vi "test.2dArrays.vi"(8 "error in":errorcluster, 10 "Data":variant, 11 "Command":string) -> (0 "error out":errorcluster, 3 "Return Data":variant)   [LabVIEW 2014]
uses:
  Private/Class/meth.Constructor.vi
  Private/Class/meth.Destructor.vi
  GLue.lvlib
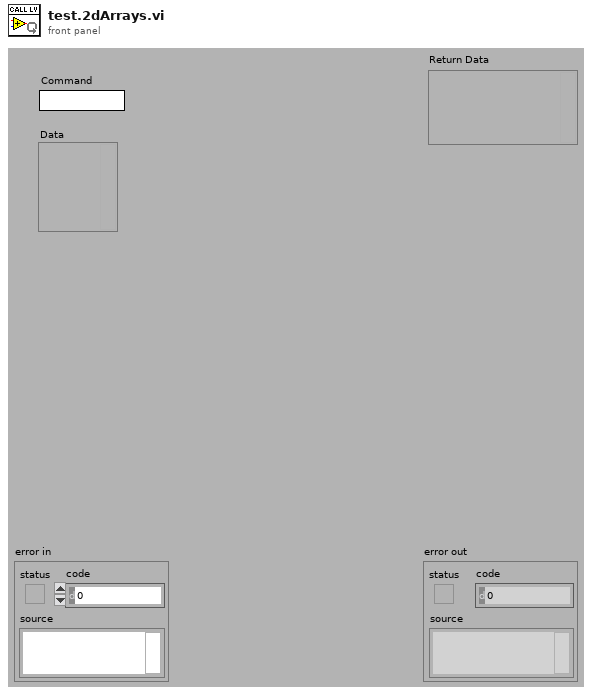
[diagram p1: front panel]
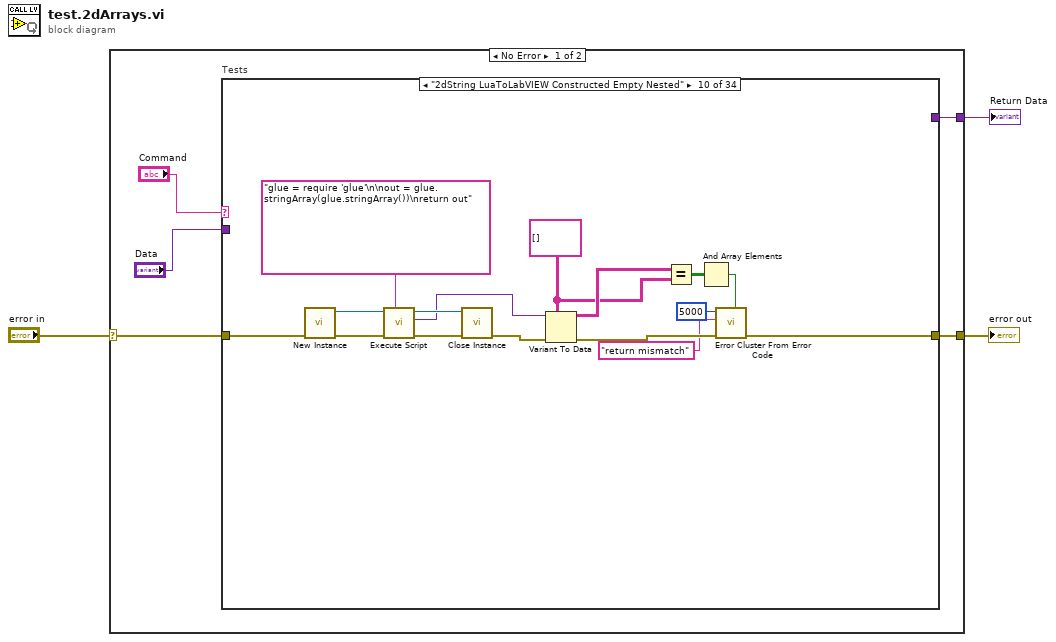
[diagram p0: block diagram]
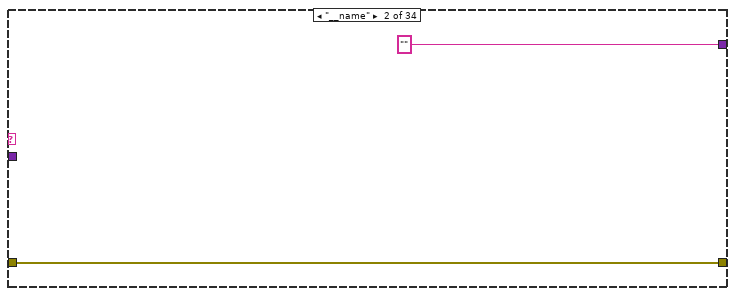
[diagram p3: hidden frame]
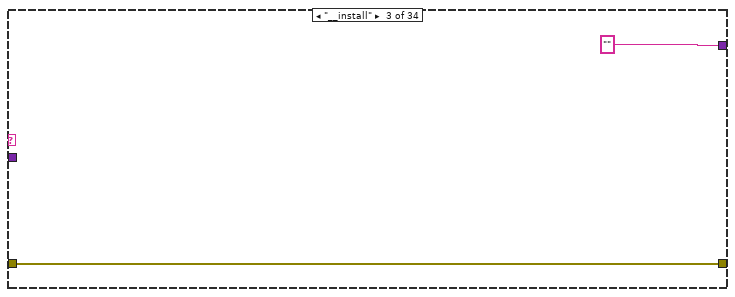
[diagram p4: hidden frame]
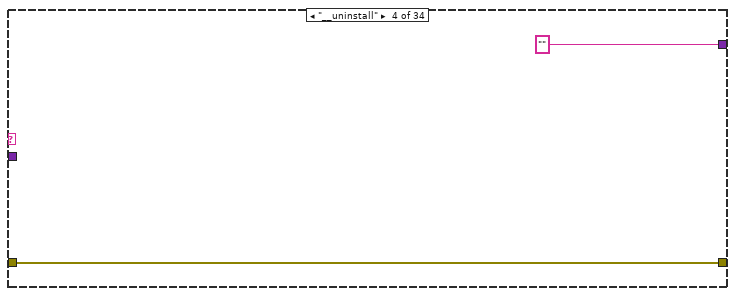
[diagram p5: hidden frame]
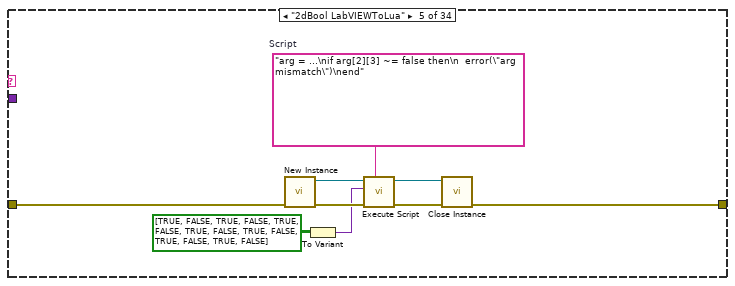
[diagram p6: hidden frame]
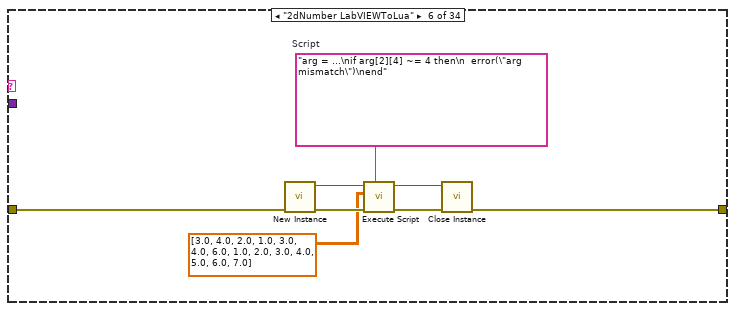
[diagram p7: hidden frame]
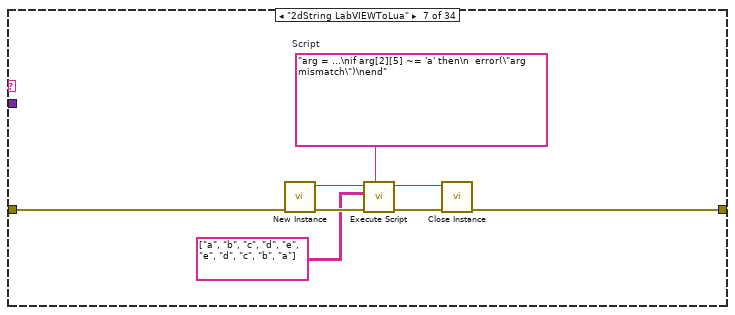
[diagram p8: hidden frame]
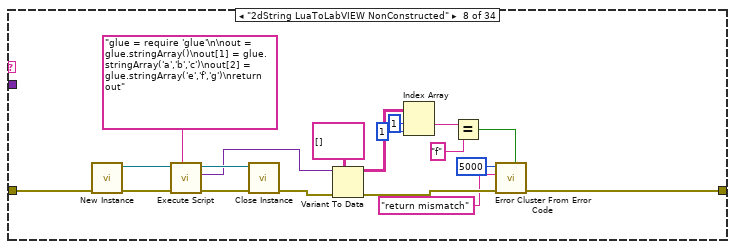
[diagram p9: hidden frame]
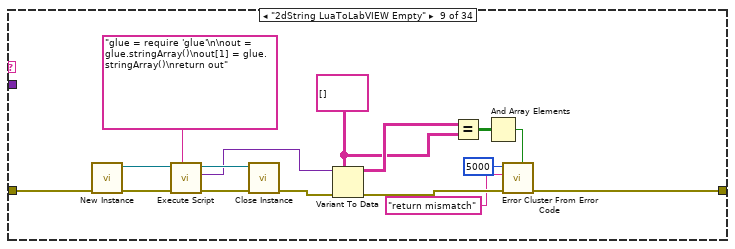
[diagram p10: hidden frame]
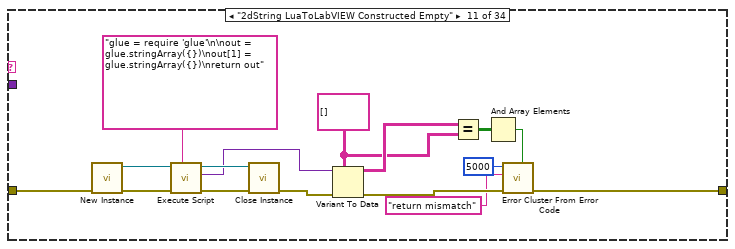
[diagram p11: hidden frame]
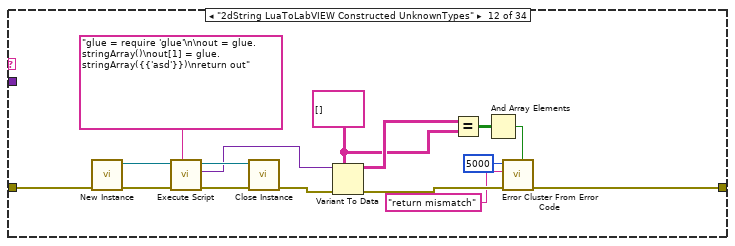
[diagram p12: hidden frame]
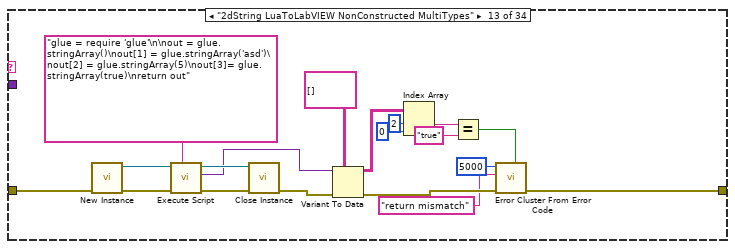
[diagram p13: hidden frame]
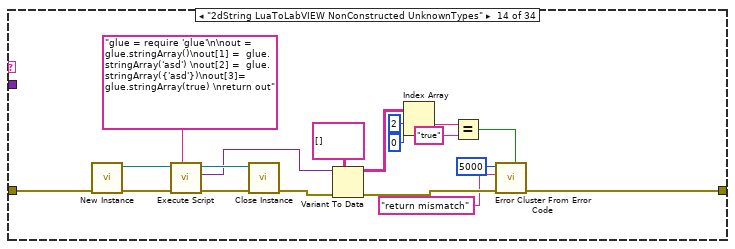
[diagram p14: hidden frame]
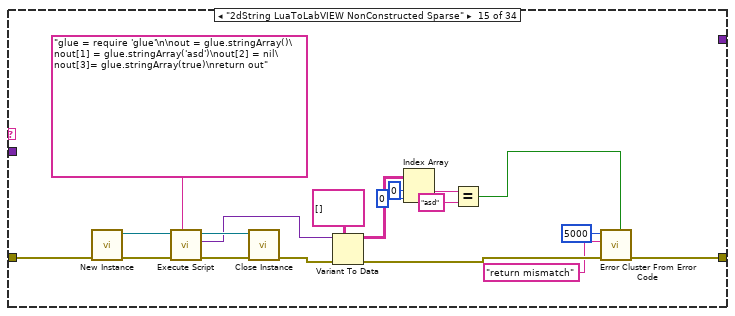
[diagram p15: hidden frame]
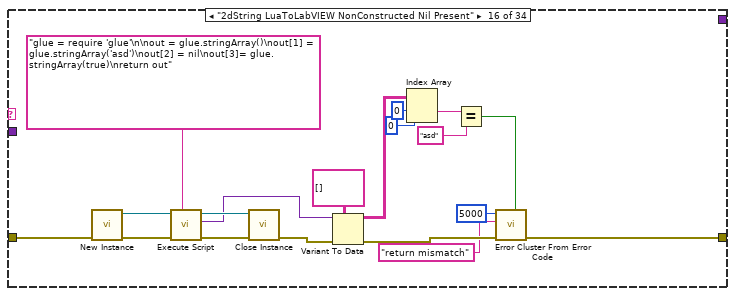
[diagram p16: hidden frame]
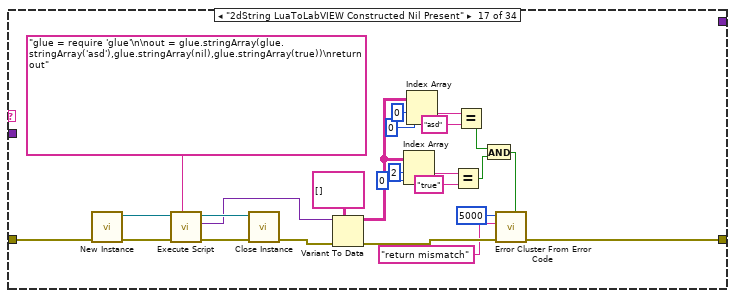
[diagram p17: hidden frame]
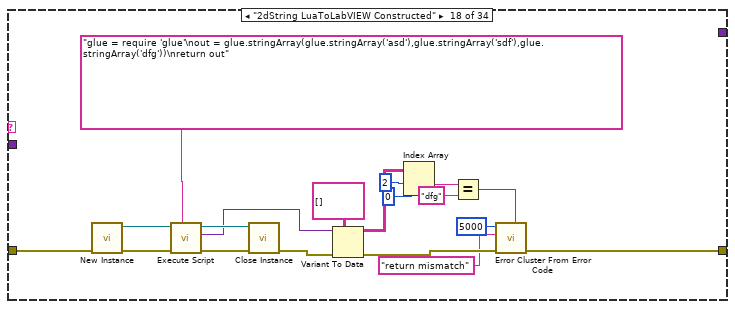
[diagram p18: hidden frame]
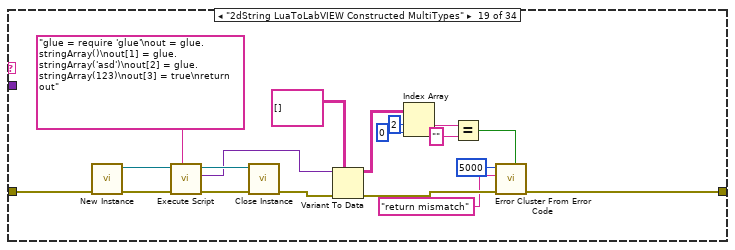
[diagram p19: hidden frame]
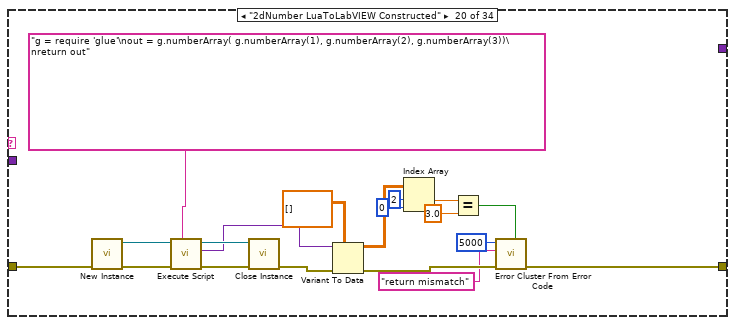
[diagram p20: hidden frame]
diagram:
  n1 = case shown="No Error" "error in" {
    selector: "error in" -> [w8 w578]
    tunnel: [w6 w578] -> w2
    tunnel: [w7 variant ("User Data")] -> w1
    frame No Error {
      n2 = case "Tests" shown="\"2dString LuaToLabVIEW Constructed Empty Nested\"" "Command" {
        tunnel: w8 -> [w10 w11 w13 w15 w20 w28 w36 w55 w71 w87 w103 w119 w138 w157 w176 w195 w220 w239 w258 w277 w296 w312 w342 w372 w398 w423 w448 w466 w483 w501 w517 w533 w552 w571]
        tunnel: "Data" -> [w9 _ _ _ _ _ _ _ _ _ _ _ _ _ _ _ _ _ _ _ _ _ _ _ _ _ _ _ _ _ _ _ _ _]
        tunnel: [w9 "" "" "" _ _ _ _ _ _ _ _ _ _ _ _ _ _ _ _ _ _ _ _ _ _ _ _ _ _ _ _ _ _] -> w7
        tunnel: [w10 w11 w13 w15 w19 w27 w35 w50 w67 w83 w99 w115 w133 w152 w171 w190 w215 w234 w253 w273 w292 w308 w338 w368 w394 w419 w444 w462 w479 w497 w513 w529 w548 w567] -> w6
        frame Default {
        }
        frame "__name" {
        }
        frame "__install" {
        }
        frame "__uninstall" {
        }
        frame "2dBool LabVIEWToLua" {
          w25 = "arg = ...\nif arg[2][3] ~= false then\n  error(\"arg mismatch\")\nend"  # Script
          n3 = call "New Instance.vi"("error in"=w20) -> ("error out"=w21:errorcluster, "GLue out"=w22:refnum<class "class.GLue.lvclass">)  [unwired: 9 in]
          n4 = To Variant(anything=bool[][] [[TRUE, FALSE, TRUE, FALSE, TRUE, FALSE, TRUE], [FALSE, TRUE, FALSE, TRUE, FALSE, TRUE, FALSE]]) -> (Variant=w17:variant)
          n5 = call "Execute Script.vi"("Script"=w25, "error in"=w21, "Argument Data"=w17, "GLue in"=w22) -> ("error out"=w23:errorcluster, "GLue out"=w24:refnum<class "class.GLue.lvclass">)  [unwired: 5 in, 1 out]
          n6 = call "Close Instance.vi"("error in"=w23, "GLue in"=w24) -> ("error out"=w19:errorcluster)  [unwired: 9 in]
        }
        frame "2dNumber LabVIEWToLua" {
          w33 = "arg = ...\nif arg[2][4] ~= 4 then\n  error(\"arg mismatch\")\nend"  # Script
          n7 = call "New Instance.vi"("error in"=w28) -> ("error out"=w29:errorcluster, "GLue out"=w30:refnum<class "class.GLue.lvclass">)  [unwired: 9 in]
          n8 = call "Execute Script.vi"("Script"=w33, "error in"=w29, "Argument Data"=dbl[][] [[3.0, 4.0, 2.0, 1.0, 3.0, 4.0, 6.0], [1.0, 2.0, 3.0, 4.0, 5.0, 6.0, 7.0]], "GLue in"=w30) -> ("error out"=w31:errorcluster, "GLue out"=w32:refnum<class "class.GLue.lvclass">)  [unwired: 5 in, 1 out]
          n9 = call "Close Instance.vi"("error in"=w31, "GLue in"=w32) -> ("error out"=w27:errorcluster)  [unwired: 9 in]
        }
        frame "2dString LabVIEWToLua" {
          w41 = "arg = ...\nif arg[2][5] ~= 'a' then\n  error(\"arg mismatch\")\nend"  # Script
          n10 = call "New Instance.vi"("error in"=w36) -> ("error out"=w37:errorcluster, "GLue out"=w38:refnum<class "class.GLue.lvclass">)  [unwired: 9 in]
          n11 = call "Execute Script.vi"("Script"=w41, "error in"=w37, "Argument Data"=string[][] [["a", "b", "c", "d", "e"], ["e", "d", "c", "b", "a"]], "GLue in"=w38) -> ("error out"=w39:errorcluster, "GLue out"=w40:refnum<class "class.GLue.lvclass">)  [unwired: 5 in, 1 out]
          n12 = call "Close Instance.vi"("error in"=w39, "GLue in"=w40) -> ("error out"=w35:errorcluster)  [unwired: 9 in]
        }
        frame "2dString LuaToLabVIEW NonConstructed" {
          n13 = call "New Instance.vi"("error in"=w55) -> ("error out"=w56:errorcluster, "GLue out"=w57:refnum<class "class.GLue.lvclass">)  [unwired: 9 in]
          n14 = call "Execute Script.vi"("Script"="glue = require 'glue'\n\nout = glue.stringArray()\nout[1] = glue.stringArray('a','b','c')\nout[2] = glue.stringArray('e','f','g')\nreturn out", "error in"=w56, "GLue in"=w57) -> ("error out"=w58:errorcluster, "Return Data"=w53:variant, "GLue out"=w59:refnum<class "class.GLue.lvclass">)  [unwired: 6 in]
          n15 = call "Close Instance.vi"("error in"=w58, "GLue in"=w59) -> ("error out"=w54:errorcluster)  [unwired: 9 in]
          n16 = Variant To Data(error in=w54, type=string[][] [], Variant=w53) -> (data=w49:string[][], error out=w51:errorcluster)
          n17 = Index Array(array=w49, index (row)=1 ("index"), index (col)=1 ("disabled index (col)")) -> (element=w47:string)
          n18 = Equal?(x=w47, y="f") -> (x = y?=w45:bool)
          n19 = call <vilib>:"Error Cluster From Error Code.vi"("is warning? (False)"=w45, "error in (no error)"=w51, "error message (\"\")"="return mismatch" ("error message (\"\")"), "error code (0)"=5000) -> ("error out"=w50:errorcluster)  [unwired: 5 in]
        }
        frame "2dString LuaToLabVIEW Empty" {
          w63 = string[][] []
          n20 = call "New Instance.vi"("error in"=w71) -> ("error out"=w72:errorcluster, "GLue out"=w73:refnum<class "class.GLue.lvclass">)  [unwired: 9 in]
          n21 = call "Execute Script.vi"("Script"="glue = require 'glue'\n\nout = glue.stringArray()\nout[1] = glue.stringArray()\nreturn out", "error in"=w72, "GLue in"=w73) -> ("error out"=w74:errorcluster, "Return Data"=w69:variant, "GLue out"=w75:refnum<class "class.GLue.lvclass">)  [unwired: 6 in]
          n22 = call "Close Instance.vi"("error in"=w74, "GLue in"=w75) -> ("error out"=w70:errorcluster)  [unwired: 9 in]
          n23 = Variant To Data(error in=w70, type=w63, Variant=w69) -> (data=w64:string[][], error out=w68:errorcluster)
          n24 = Equal?(x=w64, y=w63) -> (x = y?=w62:bool[][])
          n25 = And Array Elements(Boolean array=w62) -> (logical AND=w61:bool)
          n26 = call <vilib>:"Error Cluster From Error Code.vi"("is warning? (False)"=w61, "error in (no error)"=w68, "error message (\"\")"="return mismatch" ("error message (\"\")"), "error code (0)"=5000) -> ("error out"=w67:errorcluster)  [unwired: 5 in]
        }
        frame "2dString LuaToLabVIEW Constructed Empty Nested" {
          w79 = string[][] []
          n27 = call "New Instance.vi"("error in"=w87) -> ("error out"=w88:errorcluster, "GLue out"=w89:refnum<class "class.GLue.lvclass">)  [unwired: 9 in]
          n28 = call "Execute Script.vi"("Script"="glue = require 'glue'\n\nout = glue.stringArray(glue.stringArray())\nreturn out", "error in"=w88, "GLue in"=w89) -> ("error out"=w90:errorcluster, "Return Data"=w85:variant, "GLue out"=w91:refnum<class "class.GLue.lvclass">)  [unwired: 6 in]
          n29 = call "Close Instance.vi"("error in"=w90, "GLue in"=w91) -> ("error out"=w86:errorcluster)  [unwired: 9 in]
          n30 = Variant To Data(error in=w86, type=w79, Variant=w85) -> (data=w80:string[][], error out=w84:errorcluster)
          n31 = Equal?(x=w80, y=w79) -> (x = y?=w78:bool[][])
          n32 = And Array Elements(Boolean array=w78) -> (logical AND=w77:bool)
          n33 = call <vilib>:"Error Cluster From Error Code.vi"("is warning? (False)"=w77, "error in (no error)"=w84, "error message (\"\")"="return mismatch" ("error message (\"\")"), "error code (0)"=5000) -> ("error out"=w83:errorcluster)  [unwired: 5 in]
        }
        frame "2dString LuaToLabVIEW Constructed Empty" {
          w95 = string[][] []
          n34 = call "New Instance.vi"("error in"=w103) -> ("error out"=w104:errorcluster, "GLue out"=w105:refnum<class "class.GLue.lvclass">)  [unwired: 9 in]
          n35 = call "Execute Script.vi"("Script"="glue = require 'glue'\n\nout = glue.stringArray({})\nout[1] = glue.stringArray({})\nreturn out", "error in"=w104, "GLue in"=w105) -> ("error out"=w106:errorcluster, "Return Data"=w101:variant, "GLue out"=w107:refnum<class "class.GLue.lvclass">)  [unwired: 6 in]
          n36 = call "Close Instance.vi"("error in"=w106, "GLue in"=w107) -> ("error out"=w102:errorcluster)  [unwired: 9 in]
          n37 = Variant To Data(error in=w102, type=w95, Variant=w101) -> (data=w96:string[][], error out=w100:errorcluster)
          n38 = Equal?(x=w96, y=w95) -> (x = y?=w94:bool[][])
          n39 = And Array Elements(Boolean array=w94) -> (logical AND=w93:bool)
          n40 = call <vilib>:"Error Cluster From Error Code.vi"("is warning? (False)"=w93, "error in (no error)"=w100, "error message (\"\")"="return mismatch" ("error message (\"\")"), "error code (0)"=5000) -> ("error out"=w99:errorcluster)  [unwired: 5 in]
        }
        frame "2dString LuaToLabVIEW Constructed UnknownTypes" {
          w111 = string[][] []
          n41 = call "New Instance.vi"("error in"=w119) -> ("error out"=w120:errorcluster, "GLue out"=w121:refnum<class "class.GLue.lvclass">)  [unwired: 9 in]
          n42 = call "Execute Script.vi"("Script"="glue = require 'glue'\n\nout = glue.stringArray()\nout[1] = glue.stringArray({{'asd'}})\nreturn out", "error in"=w120, "GLue in"=w121) -> ("error out"=w122:errorcluster, "Return Data"=w117:variant, "GLue out"=w123:refnum<class "class.GLue.lvclass">)  [unwired: 6 in]
          n43 = call "Close Instance.vi"("error in"=w122, "GLue in"=w123) -> ("error out"=w118:errorcluster)  [unwired: 9 in]
          n44 = Variant To Data(error in=w118, type=w111, Variant=w117) -> (data=w112:string[][], error out=w116:errorcluster)
          n45 = Equal?(x=w112, y=w111) -> (x = y?=w110:bool[][])
          n46 = And Array Elements(Boolean array=w110) -> (logical AND=w109:bool)
          n47 = call <vilib>:"Error Cluster From Error Code.vi"("is warning? (False)"=w109, "error in (no error)"=w116, "error message (\"\")"="return mismatch" ("error message (\"\")"), "error code (0)"=5000) -> ("error out"=w115:errorcluster)  [unwired: 5 in]
        }
        frame "2dString LuaToLabVIEW NonConstructed MultiTypes" {
          n48 = call "New Instance.vi"("error in"=w138) -> ("error out"=w139:errorcluster, "GLue out"=w140:refnum<class "class.GLue.lvclass">)  [unwired: 9 in]
          n49 = call "Execute Script.vi"("Script"="glue = require 'glue'\n\nout = glue.stringArray()\nout[1] = glue.stringArray('asd')\nout[2] = glue.stringArray(5)\nout[3]= glue.stringArray(true)\nreturn out", "error in"=w139, "GLue in"=w140) -> ("error out"=w141:errorcluster, "Return Data"=w136:variant, "GLue out"=w142:refnum<class "class.GLue.lvclass">)  [unwired: 6 in]
          n50 = call "Close Instance.vi"("error in"=w141, "GLue in"=w142) -> ("error out"=w137:errorcluster)  [unwired: 9 in]
          n51 = Variant To Data(error in=w137, type=string[][] [], Variant=w136) -> (data=w132:string[][], error out=w134:errorcluster)
          n52 = Index Array(array=w132, index (row)=2 ("index"), index (col)=0 ("disabled index (col)")) -> (element=w130:string)
          n53 = Equal?(x=w130, y="true") -> (x = y?=w128:bool)
          n54 = call <vilib>:"Error Cluster From Error Code.vi"("is warning? (False)"=w128, "error in (no error)"=w134, "error message (\"\")"="return mismatch" ("error message (\"\")"), "error code (0)"=5000) -> ("error out"=w133:errorcluster)  [unwired: 5 in]
        }
        frame "2dString LuaToLabVIEW NonConstructed UnknownTypes" {
          n55 = call "New Instance.vi"("error in"=w157) -> ("error out"=w158:errorcluster, "GLue out"=w159:refnum<class "class.GLue.lvclass">)  [unwired: 9 in]
          n56 = call "Execute Script.vi"("Script"="glue = require 'glue'\n\nout = glue.stringArray()\nout[1] =  glue.stringArray('asd') \nout[2] =  glue.stringArray({'asd'})\nout[3]=  glue.stringArray(true) \nreturn out", "error in"=w158, "GLue in"=w159) -> ("error out"=w160:errorcluster, "Return Data"=w155:variant, "GLue out"=w161:refnum<class "class.GLue.lvclass">)  [unwired: 6 in]
          n57 = call "Close Instance.vi"("error in"=w160, "GLue in"=w161) -> ("error out"=w156:errorcluster)  [unwired: 9 in]
          n58 = Variant To Data(error in=w156, type=string[][] [], Variant=w155) -> (data=w151:string[][], error out=w153:errorcluster)
          n59 = Index Array(array=w151, index (row)=2 ("index"), index (col)=0 ("disabled index (col)")) -> (element=w149:string)
          n60 = Equal?(x=w149, y="true") -> (x = y?=w147:bool)
          n61 = call <vilib>:"Error Cluster From Error Code.vi"("is warning? (False)"=w147, "error in (no error)"=w153, "error message (\"\")"="return mismatch" ("error message (\"\")"), "error code (0)"=5000) -> ("error out"=w152:errorcluster)  [unwired: 5 in]
        }
        frame "2dString LuaToLabVIEW NonConstructed Sparse" {
          n62 = call "New Instance.vi"("error in"=w176) -> ("error out"=w177:errorcluster, "GLue out"=w178:refnum<class "class.GLue.lvclass">)  [unwired: 9 in]
          n63 = call "Execute Script.vi"("Script"="glue = require 'glue'\n\nout = glue.stringArray()\nout[1] = glue.stringArray('asd')\nout[2] = nil\nout[3]= glue.stringArray(true)\nreturn out", "error in"=w177, "GLue in"=w178) -> ("error out"=w179:errorcluster, "Return Data"=w174:variant, "GLue out"=w180:refnum<class "class.GLue.lvclass">)  [unwired: 6 in]
          n64 = call "Close Instance.vi"("error in"=w179, "GLue in"=w180) -> ("error out"=w175:errorcluster)  [unwired: 9 in]
          n65 = Variant To Data(error in=w175, type=string[][] [], Variant=w174) -> (data=w165:string[][], error out=w172:errorcluster)
          n66 = Index Array(array=w165, index (row)=0 ("index"), index (col)=0 ("disabled index (col)")) -> (element=w169:string)
          n67 = Equal?(x=w169, y="asd") -> (x = y?=w163:bool)
          n68 = call <vilib>:"Error Cluster From Error Code.vi"("is warning? (False)"=w163, "error in (no error)"=w172, "error message (\"\")"="return mismatch" ("error message (\"\")"), "error code (0)"=5000) -> ("error out"=w171:errorcluster)  [unwired: 5 in]
        }
        frame "2dString LuaToLabVIEW NonConstructed Nil Present" {
          n69 = call "New Instance.vi"("error in"=w195) -> ("error out"=w196:errorcluster, "GLue out"=w197:refnum<class "class.GLue.lvclass">)  [unwired: 9 in]
          n70 = call "Execute Script.vi"("Script"="glue = require 'glue'\n\nout = glue.stringArray()\nout[1] = glue.stringArray('asd')\nout[2] = nil\nout[3]= glue.stringArray(true)\nreturn out", "error in"=w196, "GLue in"=w197) -> ("error out"=w198:errorcluster, "Return Data"=w193:variant, "GLue out"=w199:refnum<class "class.GLue.lvclass">)  [unwired: 6 in]
          n71 = call "Close Instance.vi"("error in"=w198, "GLue in"=w199) -> ("error out"=w194:errorcluster)  [unwired: 9 in]
          n72 = Variant To Data(error in=w194, type=string[][] [], Variant=w193) -> (data=w184:string[][], error out=w191:errorcluster)
          n73 = Index Array(array=w184, index (row)=0 ("index"), index (col)=0 ("disabled index (col)")) -> (element=w186:string)
          n74 = Equal?(x=w186, y="asd") -> (x = y?=w182:bool)
          n75 = call <vilib>:"Error Cluster From Error Code.vi"("is warning? (False)"=w182, "error in (no error)"=w191, "error message (\"\")"="return mismatch" ("error message (\"\")"), "error code (0)"=5000) -> ("error out"=w190:errorcluster)  [unwired: 5 in]
        }
        frame "2dString LuaToLabVIEW Constructed Nil Present" {
          n76 = call "New Instance.vi"("error in"=w220) -> ("error out"=w221:errorcluster, "GLue out"=w222:refnum<class "class.GLue.lvclass">)  [unwired: 9 in]
          n77 = call "Execute Script.vi"("Script"="glue = require 'glue'\n\nout = glue.stringArray(glue.stringArray('asd'),glue.stringArray(nil),glue.stringArray(true))\nreturn out", "error in"=w221, "GLue in"=w222) -> ("error out"=w223:errorcluster, "Return Data"=w218:variant, "GLue out"=w224:refnum<class "class.GLue.lvclass">)  [unwired: 6 in]
          n78 = call "Close Instance.vi"("error in"=w223, "GLue in"=w224) -> ("error out"=w219:errorcluster)  [unwired: 9 in]
          n79 = Variant To Data(error in=w219, type=string[][] [], Variant=w218) -> (data=w207:string[][], error out=w216:errorcluster)
          n80 = Index Array(array=w207, index (row)=2 ("index"), index (col)=0 ("disabled index (col)")) -> (element=w213:string)
          n81 = Index Array(array=w207, index (row)=0 ("index"), index (col)=0 ("disabled index (col)")) -> (element=w209:string)
          n82 = Equal?(x=w213, y="true") -> (x = y?=w205:bool)
          n83 = Equal?(x=w209, y="asd") -> (x = y?=w206:bool)
          n84 = And(x=w206, y=w205) -> (x .and. y?=w204:bool)
          n85 = call <vilib>:"Error Cluster From Error Code.vi"("is warning? (False)"=w204, "error in (no error)"=w216, "error message (\"\")"="return mismatch" ("error message (\"\")"), "error code (0)"=5000) -> ("error out"=w215:errorcluster)  [unwired: 5 in]
        }
        frame "2dString LuaToLabVIEW Constructed" {
          n86 = call "New Instance.vi"("error in"=w239) -> ("error out"=w240:errorcluster, "GLue out"=w241:refnum<class "class.GLue.lvclass">)  [unwired: 9 in]
          n87 = call "Execute Script.vi"("Script"="glue = require 'glue'\nout = glue.stringArray(glue.stringArray('asd'),glue.stringArray('sdf'),glue.stringArray('dfg'))\nreturn out", "error in"=w240, "GLue in"=w241) -> ("error out"=w242:errorcluster, "Return Data"=w237:variant, "GLue out"=w243:refnum<class "class.GLue.lvclass">)  [unwired: 6 in]
          n88 = call "Close Instance.vi"("error in"=w242, "GLue in"=w243) -> ("error out"=w238:errorcluster)  [unwired: 9 in]
          n89 = Variant To Data(error in=w238, type=string[][] [], Variant=w237) -> (data=w233:string[][], error out=w235:errorcluster)
          n90 = Index Array(array=w233, index (row)=2 ("index"), index (col)=0 ("disabled index (col)")) -> (element=w231:string)
          n91 = Equal?(x=w231, y="dfg") -> (x = y?=w229:bool)
          n92 = call <vilib>:"Error Cluster From Error Code.vi"("is warning? (False)"=w229, "error in (no error)"=w235, "error message (\"\")"="return mismatch" ("error message (\"\")"), "error code (0)"=5000) -> ("error out"=w234:errorcluster)  [unwired: 5 in]
        }
        frame "2dString LuaToLabVIEW Constructed MultiTypes" {
          n93 = call "New Instance.vi"("error in"=w258) -> ("error out"=w259:errorcluster, "GLue out"=w260:refnum<class "class.GLue.lvclass">)  [unwired: 9 in]
          n94 = call "Execute Script.vi"("Script"="glue = require 'glue'\nout = glue.stringArray()\nout[1] = glue.stringArray('asd')\nout[2] = glue.stringArray(123)\nout[3] = true\nreturn out", "error in"=w259, "GLue in"=w260) -> ("error out"=w261:errorcluster, "Return Data"=w256:variant, "GLue out"=w262:refnum<class "class.GLue.lvclass">)  [unwired: 6 in]
          n95 = call "Close Instance.vi"("error in"=w261, "GLue in"=w262) -> ("error out"=w257:errorcluster)  [unwired: 9 in]
          n96 = Variant To Data(error in=w257, type=string[][] [], Variant=w256) -> (data=w252:string[][], error out=w254:errorcluster)
          n97 = Index Array(array=w252, index (row)=2 ("index"), index (col)=0 ("disabled index (col)")) -> (element=w250:string)
          n98 = Equal?(x=w250, y="") -> (x = y?=w248:bool)
          n99 = call <vilib>:"Error Cluster From Error Code.vi"("is warning? (False)"=w248, "error in (no error)"=w254, "error message (\"\")"="return mismatch" ("error message (\"\")"), "error code (0)"=5000) -> ("error out"=w253:errorcluster)  [unwired: 5 in]
        }
        frame "2dNumber LuaToLabVIEW Constructed" {
          n100 = call "New Instance.vi"("error in"=w277) -> ("error out"=w278:errorcluster, "GLue out"=w279:refnum<class "class.GLue.lvclass">)  [unwired: 9 in]
          n101 = call "Execute Script.vi"("Script"="g = require 'glue'\nout = g.numberArray( g.numberArray(1), g.numberArray(2), g.numberArray(3))\nreturn out", "error in"=w278, "GLue in"=w279) -> ("error out"=w280:errorcluster, "Return Data"=w275:variant, "GLue out"=w281:refnum<class "class.GLue.lvclass">)  [unwired: 6 in]
          n102 = call "Close Instance.vi"("error in"=w280, "GLue in"=w281) -> ("error out"=w276:errorcluster)  [unwired: 9 in]
          n103 = Variant To Data(error in=w276, type=dbl[][] [], Variant=w275) -> (data=w272:dbl[][], error out=w274:errorcluster)
          n104 = Index Array(array=w272, index (row)=2 ("index"), index (col)=0 ("disabled index (col)")) -> (element=w270:dbl)
          n105 = Equal?(x=w270, y=3.0) -> (x = y?=w269:bool)
          n106 = call <vilib>:"Error Cluster From Error Code.vi"("is warning? (False)"=w269, "error in (no error)"=w274, "error message (\"\")"="return mismatch" ("error message (\"\")"), "error code (0)"=5000) -> ("error out"=w273:errorcluster)  [unwired: 5 in]
        }
        frame "2dNumber LuaToLabVIEW Constructed Nil Present" {
          n107 = call "New Instance.vi"("error in"=w296) -> ("error out"=w297:errorcluster, "GLue out"=w298:refnum<class "class.GLue.lvclass">)  [unwired: 9 in]
          n108 = call "Execute Script.vi"("Script"="g = require 'glue'\nout = g.numberArray( g.numberArray(1), nil, g.numberArray(3))\nreturn out", "error in"=w297, "GLue in"=w298) -> ("error out"=w299:errorcluster, "Return Data"=w294:variant, "GLue out"=w300:refnum<class "class.GLue.lvclass">)  [unwired: 6 in]
          n109 = call "Close Instance.vi"("error in"=w299, "GLue in"=w300) -> ("error out"=w295:errorcluster)  [unwired: 9 in]
          n110 = Variant To Data(error in=w295, type=dbl[][] [], Variant=w294) -> (data=w291:dbl[][], error out=w293:errorcluster)
          n111 = Index Array(array=w291, index (row)=2 ("index"), index (col)=0 ("disabled index (col)")) -> (element=w289:dbl)
          n112 = Equal?(x=w289, y=3.0) -> (x = y?=w288:bool)
          n113 = call <vilib>:"Error Cluster From Error Code.vi"("is warning? (False)"=w288, "error in (no error)"=w293, "error message (\"\")"="return mismatch" ("error message (\"\")"), "error code (0)"=5000) -> ("error out"=w292:errorcluster)  [unwired: 5 in]
        }
        frame "2dNumber LuaToLabVIEW Constructed Empty" {
          w304 = dbl[][] []
          n114 = call "New Instance.vi"("error in"=w312) -> ("error out"=w313:errorcluster, "GLue out"=w314:refnum<class "class.GLue.lvclass">)  [unwired: 9 in]
          n115 = call "Execute Script.vi"("Script"="glue = require 'glue'\nout = glue.numberArray( glue.numberArray())\nreturn out", "error in"=w313, "GLue in"=w314) -> ("error out"=w315:errorcluster, "Return Data"=w310:variant, "GLue out"=w316:refnum<class "class.GLue.lvclass">)  [unwired: 6 in]
          n116 = call "Close Instance.vi"("error in"=w315, "GLue in"=w316) -> ("error out"=w311:errorcluster)  [unwired: 9 in]
          n117 = Variant To Data(error in=w311, type=w304, Variant=w310) -> (data=w305:dbl[][], error out=w309:errorcluster)
          n118 = Equal?(x=w305, y=w304) -> (x = y?=w303:bool[][])
          n119 = And Array Elements(Boolean array=w303) -> (logical AND=w302:bool)
          n120 = call <vilib>:"Error Cluster From Error Code.vi"("is warning? (False)"=w302, "error in (no error)"=w309, "error message (\"\")"="return mismatch" ("error message (\"\")"), "error code (0)"=5000) -> ("error out"=w308:errorcluster)  [unwired: 5 in]
        }
        frame "2dNumber LuaToLabVIEW Constructed MultiTypes" {
          n121 = call "New Instance.vi"("error in"=w342) -> ("error out"=w343:errorcluster, "GLue out"=w344:refnum<class "class.GLue.lvclass">)  [unwired: 9 in]
          n122 = call "Execute Script.vi"("Script"="g = require 'glue'\nout = g.numberArray(g.numberArray(1),g.numberArray('asd'),g.numberArray(true),g.numberArray(nil))\nreturn out", "error in"=w343, "GLue in"=w344) -> ("error out"=w345:errorcluster, "Return Data"=w340:variant, "GLue out"=w346:refnum<class "class.GLue.lvclass">)  [unwired: 6 in]
          n123 = call "Close Instance.vi"("error in"=w345, "GLue in"=w346) -> ("error out"=w341:errorcluster)  [unwired: 9 in]
          n124 = Variant To Data(error in=w341, type=dbl[][] [], Variant=w340) -> (data=w322:dbl[][], error out=w339:errorcluster)
          n125 = Index Array(array=w322, index (row)=0 ("index"), index (col)=0 ("disabled index (col)")) -> (element=w336:dbl)
          n126 = Index Array(array=w322, index (row)=3 ("index"), index (col)=0 ("disabled index (col)")) -> (element=w330:dbl)
          n127 = Index Array(array=w322, index (row)=3 ("index"), index (col)=0 ("disabled index (col)")) -> (element=w324:dbl)
          n128 = Equal?(x=w336, y=1.0) -> (x = y?=w327:bool)
          n129 = Equal?(x=w330, y=0.0) -> (x = y?=w328:bool)
          n130 = Equal?(x=w324, y=0.0) -> (x = y?=w321:bool)
          n131 = Compound Arithmetic op=AND(w321, w328, w327) -> (w326:bool)
          n132 = call <vilib>:"Error Cluster From Error Code.vi"("is warning? (False)"=w326, "error in (no error)"=w339, "error message (\"\")"="return mismatch" ("error message (\"\")"), "error code (0)"=5000) -> ("error out"=w338:errorcluster)  [unwired: 5 in]
        }
        frame "2dNumber LuaToLabVIEW NonConstructed MultiTypes" {
          n133 = call "New Instance.vi"("error in"=w372) -> ("error out"=w373:errorcluster, "GLue out"=w374:refnum<class "class.GLue.lvclass">)  [unwired: 9 in]
          n134 = call "Execute Script.vi"("Script"="glue = require 'glue'\nout = glue.numberArray()\nout[1] = glue.numberArray(1)\nout[2] = glue.numberArray('asd')\nout[3] = glue.numberArray(true)\nout[4] = glue.numberArray(2)\nreturn out", "error in"=w373, "GLue in"=w374) -> ("error out"=w375:errorcluster, "Return Data"=w370:variant, "GLue out"=w376:refnum<class "class.GLue.lvclass">)  [unwired: 6 in]
          n135 = call "Close Instance.vi"("error in"=w375, "GLue in"=w376) -> ("error out"=w371:errorcluster)  [unwired: 9 in]
          n136 = Variant To Data(error in=w371, type=dbl[][] [], Variant=w370) -> (data=w352:dbl[][], error out=w369:errorcluster)
          n137 = Index Array(array=w352, index (row)=0 ("index"), index (col)=0 ("disabled index (col)")) -> (element=w366:dbl)
          n138 = Index Array(array=w352, index (row)=3 ("index"), index (col)=0 ("disabled index (col)")) -> (element=w360:dbl)
          n139 = Index Array(array=w352, index (row)=1 ("index"), index (col)=0 ("disabled index (col)")) -> (element=w354:dbl)
          n140 = Equal?(x=w366, y=1.0) -> (x = y?=w357:bool)
          n141 = Equal?(x=w360, y=2.0) -> (x = y?=w358:bool)
          n142 = Equal?(x=w354, y=0.0) -> (x = y?=w351:bool)
          n143 = Compound Arithmetic op=AND(w351, w358, w357) -> (w356:bool)
          n144 = call <vilib>:"Error Cluster From Error Code.vi"("is warning? (False)"=w356, "error in (no error)"=w369, "error message (\"\")"="return mismatch" ("error message (\"\")"), "error code (0)"=5000) -> ("error out"=w368:errorcluster)  [unwired: 5 in]
        }
        frame "2dBool LuaToLabVIEW NonConstructed" {
          n145 = call "New Instance.vi"("error in"=w398) -> ("error out"=w399:errorcluster, "GLue out"=w400:refnum<class "class.GLue.lvclass">)  [unwired: 9 in]
          n146 = call "Execute Script.vi"("Script"="glue = require 'glue'\nout = glue.boolArray()\nout[1] = glue.boolArray(false)\nout[2] = glue.boolArray(true)\nout[3] = glue.boolArray(true)\nout[4] = glue.boolArray(false)\nreturn out", "error in"=w399, "GLue in"=w400) -> ("error out"=w401:errorcluster, "Return Data"=w396:variant, "GLue out"=w402:refnum<class "class.GLue.lvclass">)  [unwired: 6 in]
          n147 = call "Close Instance.vi"("error in"=w401, "GLue in"=w402) -> ("error out"=w397:errorcluster)  [unwired: 9 in]
          n148 = Variant To Data(error in=w397, type=bool[][] [], Variant=w396) -> (data=w386:bool[][], error out=w395:errorcluster)
          n149 = Index Array(array=w386, index (row)=0 ("index"), index (col)=0 ("disabled index (col)")) -> (element=w385:bool)
          n150 = Index Array(array=w386, index (row)=3 ("index"), index (col)=0 ("disabled index (col)")) -> (element=w384:bool)
          n151 = Index Array(array=w386, index (row)=1 ("index"), index (col)=0 ("disabled index (col)")) -> (element=w383:bool)
          n152 = Not(x=w384) -> (.not. x?=w382:bool)
          n153 = Not(x=w385) -> (.not. x?=w381:bool)
          n154 = Compound Arithmetic op=AND(w383, w382, w381) -> (w388:bool)
          n155 = call <vilib>:"Error Cluster From Error Code.vi"("is warning? (False)"=w388, "error in (no error)"=w395, "error message (\"\")"="return mismatch" ("error message (\"\")"), "error code (0)"=5000) -> ("error out"=w394:errorcluster)  [unwired: 5 in]
        }
        frame "2dBool LuaToLabVIEW NonConstructed MultiTypes" {
          n156 = call "New Instance.vi"("error in"=w423) -> ("error out"=w424:errorcluster, "GLue out"=w425:refnum<class "class.GLue.lvclass">)  [unwired: 9 in]
          n157 = call "Execute Script.vi"("Script"="glue = require 'glue'\nout = glue.boolArray()\nout[1] = glue.boolArray(false)\nout[2] = glue.boolArray(5)\nout[3] = glue.boolArray('false')\nreturn out", "error in"=w424, "GLue in"=w425) -> ("error out"=w426:errorcluster, "Return Data"=w421:variant, "GLue out"=w427:refnum<class "class.GLue.lvclass">)  [unwired: 6 in]
          n158 = call "Close Instance.vi"("error in"=w426, "GLue in"=w427) -> ("error out"=w422:errorcluster)  [unwired: 9 in]
          n159 = Variant To Data(error in=w422, type=bool[][] [], Variant=w421) -> (data=w411:bool[][], error out=w420:errorcluster)
          n160 = Index Array(array=w411, index (row)=0 ("index"), index (col)=0 ("disabled index (col)")) -> (element=w410:bool)
          n161 = Index Array(array=w411, index (row)=1 ("index"), index (col)=0 ("disabled index (col)")) -> (element=w407:bool)
          n162 = Index Array(array=w411, index (row)=2 ("index"), index (col)=0 ("disabled index (col)")) -> (element=w409:bool)
          n163 = Not(x=w410) -> (.not. x?=w408:bool)
          n164 = Compound Arithmetic op=AND(w409, w407, w408) -> (w413:bool)
          n165 = call <vilib>:"Error Cluster From Error Code.vi"("is warning? (False)"=w413, "error in (no error)"=w420, "error message (\"\")"="return mismatch" ("error message (\"\")"), "error code (0)"=5000) -> ("error out"=w419:errorcluster)  [unwired: 5 in]
        }
        frame "2dBool LuaToLabVIEW Constructed MultiTypes" {
          n166 = call "New Instance.vi"("error in"=w448) -> ("error out"=w449:errorcluster, "GLue out"=w450:refnum<class "class.GLue.lvclass">)  [unwired: 9 in]
          n167 = call "Execute Script.vi"("Script"="glue = require 'glue'\nout = glue.boolArray(glue.boolArray(false),glue.boolArray(5),glue.boolArray('test'))\nreturn out", "error in"=w449, "GLue in"=w450) -> ("error out"=w451:errorcluster, "Return Data"=w446:variant, "GLue out"=w452:refnum<class "class.GLue.lvclass">)  [unwired: 6 in]
          n168 = call "Close Instance.vi"("error in"=w451, "GLue in"=w452) -> ("error out"=w447:errorcluster)  [unwired: 9 in]
          n169 = Variant To Data(error in=w447, type=bool[][] [], Variant=w446) -> (data=w436:bool[][], error out=w445:errorcluster)
          n170 = Index Array(array=w436, index (row)=0 ("index"), index (col)=0 ("disabled index (col)")) -> (element=w435:bool)
          n171 = Index Array(array=w436, index (row)=1 ("index"), index (col)=0 ("disabled index (col)")) -> (element=w432:bool)
          n172 = Index Array(array=w436, index (row)=2 ("index"), index (col)=0 ("disabled index (col)")) -> (element=w434:bool)
          n173 = Not(x=w435) -> (.not. x?=w433:bool)
          n174 = Compound Arithmetic op=AND(w434, w432, w433) -> (w438:bool)
          n175 = call <vilib>:"Error Cluster From Error Code.vi"("is warning? (False)"=w438, "error in (no error)"=w445, "error message (\"\")"="return mismatch" ("error message (\"\")"), "error code (0)"=5000) -> ("error out"=w444:errorcluster)  [unwired: 5 in]
        }
        frame "2dBool LuaToLabVIEW NonConstructed Sparse" {
          n176 = call "New Instance.vi"("error in"=w466) -> ("error out"=w467:errorcluster, "GLue out"=w468:refnum<class "class.GLue.lvclass">)  [unwired: 9 in]
          n177 = call "Execute Script.vi"("Script"="glue = require 'glue'\nout = glue.boolArray()\nout[1] = glue.boolArray(true)\nout[2] = nil\nout[3] = glue.boolArray(true)\nreturn out", "error in"=w467, "GLue in"=w468) -> ("error out"=w469:errorcluster, "Return Data"=w464:variant, "GLue out"=w470:refnum<class "class.GLue.lvclass">)  [unwired: 6 in]
          n178 = call "Close Instance.vi"("error in"=w469, "GLue in"=w470) -> ("error out"=w465:errorcluster)  [unwired: 9 in]
          n179 = Variant To Data(error in=w465, type=bool[][] [], Variant=w464) -> (data=w457:bool[][], error out=w463:errorcluster)
          n180 = Index Array(array=w457, index (row)=2 ("index"), index (col)=0 ("disabled index (col)")) -> (element=w455:bool)
          n181 = Not(x=w455) -> (.not. x?=w454:bool)
          n182 = call <vilib>:"Error Cluster From Error Code.vi"("is warning? (False)"=w454, "error in (no error)"=w463, "error message (\"\")"="return mismatch" ("error message (\"\")"), "error code (0)"=5000) -> ("error out"=w462:errorcluster)  [unwired: 5 in]
        }
        frame "2dBool LuaToLabVIEW Constructed Nil Present" {
          n183 = call "New Instance.vi"("error in"=w483) -> ("error out"=w484:errorcluster, "GLue out"=w485:refnum<class "class.GLue.lvclass">)  [unwired: 9 in]
          n184 = call "Execute Script.vi"("Script"="g = require 'glue'\nout = g.boolArray(g.boolArray(true),g.boolArray(nil),g.boolArray(true))\nreturn out", "error in"=w484, "GLue in"=w485) -> ("error out"=w486:errorcluster, "Return Data"=w481:variant, "GLue out"=w487:refnum<class "class.GLue.lvclass">)  [unwired: 6 in]
          n185 = call "Close Instance.vi"("error in"=w486, "GLue in"=w487) -> ("error out"=w482:errorcluster)  [unwired: 9 in]
          n186 = Variant To Data(error in=w482, type=bool[][] [], Variant=w481) -> (data=w474:bool[][], error out=w480:errorcluster)
          n187 = Index Array(array=w474, index (row)=2 ("index"), index (col)=0 ("disabled index (col)")) -> (element=w472:bool)
          n188 = call <vilib>:"Error Cluster From Error Code.vi"("is warning? (False)"=w472, "error in (no error)"=w480, "error message (\"\")"="return mismatch" ("error message (\"\")"), "error code (0)"=5000) -> ("error out"=w479:errorcluster)  [unwired: 5 in]
        }
        frame "2dBool LuaToLabVIEW NonConstructed Nil Present" {
          n189 = call "New Instance.vi"("error in"=w501) -> ("error out"=w502:errorcluster, "GLue out"=w503:refnum<class "class.GLue.lvclass">)  [unwired: 9 in]
          n190 = call "Execute Script.vi"("Script"="g = require 'glue'\nout = g.boolArray()\nout[1] = g.boolArray(false)\nout[2] = g.boolArray(nil)\nout[3] = g.boolArray('true')\nreturn out", "error in"=w502, "GLue in"=w503) -> ("error out"=w504:errorcluster, "Return Data"=w499:variant, "GLue out"=w505:refnum<class "class.GLue.lvclass">)  [unwired: 6 in]
          n191 = call "Close Instance.vi"("error in"=w504, "GLue in"=w505) -> ("error out"=w500:errorcluster)  [unwired: 9 in]
          n192 = Variant To Data(error in=w500, type=bool[][] [], Variant=w499) -> (data=w492:bool[][], error out=w498:errorcluster)
          n193 = Index Array(array=w492, index (row)=0 ("index"), index (col)=0 ("disabled index (col)")) -> (element=w490:bool)
          n194 = Not(x=w490) -> (.not. x?=w489:bool)
          n195 = call <vilib>:"Error Cluster From Error Code.vi"("is warning? (False)"=w489, "error in (no error)"=w498, "error message (\"\")"="return mismatch" ("error message (\"\")"), "error code (0)"=5000) -> ("error out"=w497:errorcluster)  [unwired: 5 in]
        }
        frame "2dBool LuaToLabVIEW NonConstructed Empty" {
          w509 = bool[][] []
          n196 = call "New Instance.vi"("error in"=w517) -> ("error out"=w518:errorcluster, "GLue out"=w519:refnum<class "class.GLue.lvclass">)  [unwired: 9 in]
          n197 = call "Execute Script.vi"("Script"="glue = require 'glue'\nout = glue.boolArray()\nout[1] = glue.boolArray()\nreturn out", "error in"=w518, "GLue in"=w519) -> ("error out"=w520:errorcluster, "Return Data"=w515:variant, "GLue out"=w521:refnum<class "class.GLue.lvclass">)  [unwired: 6 in]
          n198 = call "Close Instance.vi"("error in"=w520, "GLue in"=w521) -> ("error out"=w516:errorcluster)  [unwired: 9 in]
          n199 = Variant To Data(error in=w516, type=w509, Variant=w515) -> (data=w510:bool[][], error out=w514:errorcluster)
          n200 = Equal?(x=w510, y=w509) -> (x = y?=w508:bool[][])
          n201 = And Array Elements(Boolean array=w508) -> (logical AND=w507:bool)
          n202 = call <vilib>:"Error Cluster From Error Code.vi"("is warning? (False)"=w507, "error in (no error)"=w514, "error message (\"\")"="return mismatch" ("error message (\"\")"), "error code (0)"=5000) -> ("error out"=w513:errorcluster)  [unwired: 5 in]
        }
        frame "2dBool LuaToLabVIEW Constructed Empty" {
          w525 = bool[][] []
          n203 = call "New Instance.vi"("error in"=w533) -> ("error out"=w534:errorcluster, "GLue out"=w535:refnum<class "class.GLue.lvclass">)  [unwired: 9 in]
          n204 = call "Execute Script.vi"("Script"="glue = require 'glue'\nout = glue.boolArray(glue.boolArray())\nreturn out", "error in"=w534, "GLue in"=w535) -> ("error out"=w536:errorcluster, "Return Data"=w531:variant, "GLue out"=w537:refnum<class "class.GLue.lvclass">)  [unwired: 6 in]
          n205 = call "Close Instance.vi"("error in"=w536, "GLue in"=w537) -> ("error out"=w532:errorcluster)  [unwired: 9 in]
          n206 = Variant To Data(error in=w532, type=w525, Variant=w531) -> (data=w526:bool[][], error out=w530:errorcluster)
          n207 = Equal?(x=w526, y=w525) -> (x = y?=w524:bool[][])
          n208 = And Array Elements(Boolean array=w524) -> (logical AND=w523:bool)
          n209 = call <vilib>:"Error Cluster From Error Code.vi"("is warning? (False)"=w523, "error in (no error)"=w530, "error message (\"\")"="return mismatch" ("error message (\"\")"), "error code (0)"=5000) -> ("error out"=w529:errorcluster)  [unwired: 5 in]
        }
        frame "2dNumber LuaToLabVIEW NonConstructed Sparse" {
          n210 = call "New Instance.vi"("error in"=w552) -> ("error out"=w553:errorcluster, "GLue out"=w554:refnum<class "class.GLue.lvclass">)  [unwired: 9 in]
          n211 = call "Execute Script.vi"("Script"="glue = require 'glue'\nout = glue.numberArray()\nout[1] = glue.numberArray(1)\nout[2] = nil\nout[3] = glue.numberArray(3)\nreturn out", "error in"=w553, "GLue in"=w554) -> ("error out"=w555:errorcluster, "Return Data"=w550:variant, "GLue out"=w556:refnum<class "class.GLue.lvclass">)  [unwired: 6 in]
          n212 = call "Close Instance.vi"("error in"=w555, "GLue in"=w556) -> ("error out"=w551:errorcluster)  [unwired: 9 in]
          n213 = Variant To Data(error in=w551, type=dbl[][] [], Variant=w550) -> (data=w541:dbl[][], error out=w549:errorcluster)
          n214 = Index Array(array=w541, index (row)=0 ("index"), index (col)=0 ("disabled index (col)")) -> (element=w546:dbl)
          n215 = Equal?(x=w546, y=1.0) -> (x = y?=w539:bool)
          n216 = call <vilib>:"Error Cluster From Error Code.vi"("is warning? (False)"=w539, "error in (no error)"=w549, "error message (\"\")"="return mismatch" ("error message (\"\")"), "error code (0)"=5000) -> ("error out"=w548:errorcluster)  [unwired: 5 in]
        }
        frame "2dNumber LuaToLabVIEW NonConstructed Nil Present" {
          n217 = call "New Instance.vi"("error in"=w571) -> ("error out"=w572:errorcluster, "GLue out"=w573:refnum<class "class.GLue.lvclass">)  [unwired: 9 in]
          n218 = call "Execute Script.vi"("Script"="glue = require 'glue'\nout = glue.numberArray()\nout[1] = glue.numberArray(1)\nout[2] = glue.numberArray('asd')\nout[3] = nil\nout[4] = glue.numberArray(2)\nreturn out", "error in"=w572, "GLue in"=w573) -> ("error out"=w574:errorcluster, "Return Data"=w569:variant, "GLue out"=w575:refnum<class "class.GLue.lvclass">)  [unwired: 6 in]
          n219 = call "Close Instance.vi"("error in"=w574, "GLue in"=w575) -> ("error out"=w570:errorcluster)  [unwired: 9 in]
          n220 = Variant To Data(error in=w570, type=dbl[][] [], Variant=w569) -> (data=w560:dbl[][], error out=w568:errorcluster)
          n221 = Index Array(array=w560, index (row)=0 ("index"), index (col)=0 ("disabled index (col)")) -> (element=w565:dbl)
          n222 = Equal?(x=w565, y=1.0) -> (x = y?=w558:bool)
          n223 = call <vilib>:"Error Cluster From Error Code.vi"("is warning? (False)"=w558, "error in (no error)"=w568, "error message (\"\")"="return mismatch" ("error message (\"\")"), "error code (0)"=5000) -> ("error out"=w567:errorcluster)  [unwired: 5 in]
        }
      }
    }
    frame Error {
    }
  }
  "Return Data" <- w1
  "error out" <- w2
